vi "Rozdziel_na_Syg_typ.vi"(6 "Property Syg_typ":string[](array[string]), 8 "error in (no error)":errorcluster, 9 "data":waveform(dbl)[](array[waveform])) -> (0 "error out":errorcluster, 3 "Przebiegi":T1)   [LabVIEW 2014]
doc: "Rozdziela przebiegi wczytane z pliku TDMS\nna typy Analogowy, Cyfrowy i enkoderowy\ndla okna edycji, zgodnie z typedef Kanaly.ctl"
uses:
  Kontrolki/Przetwarzanie/Kanaly.ctl
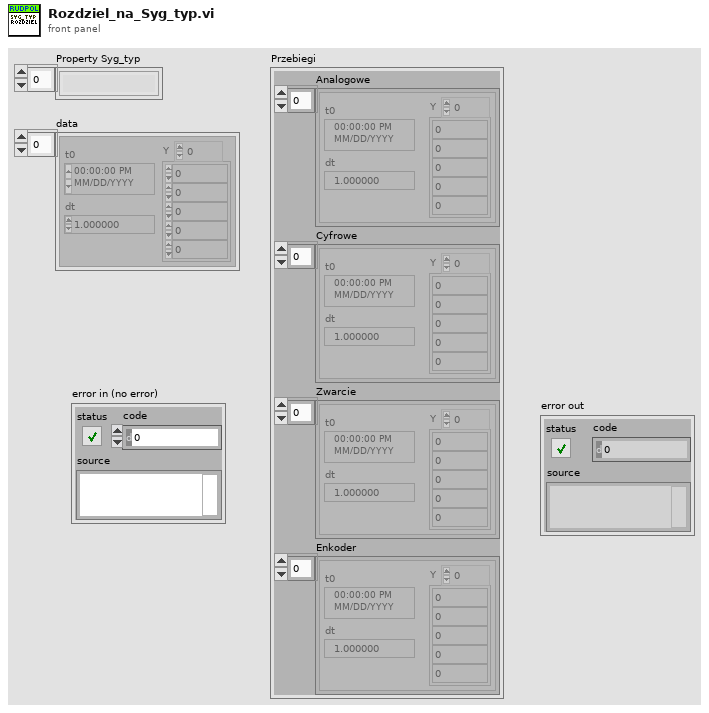
[diagram p1: front panel]
types:
  T1 = typedef "Kanaly.ctl" = cluster{"Analogowe":waveform(dbl)[], "Cyfrowe":waveform(dbl)[], "Zwarcie":waveform(dbl)[], "Enkoder":waveform(dbl)[]}
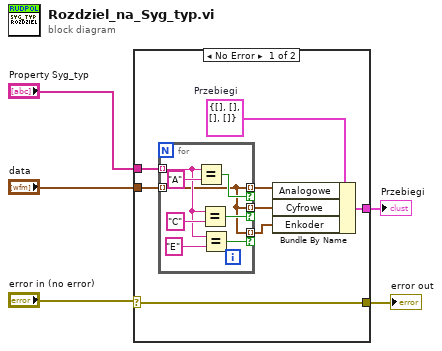
[diagram p0: block diagram]
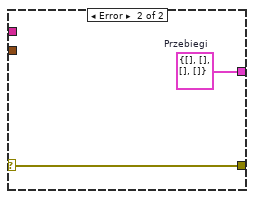
[diagram p2: hidden frame]
diagram:
  n1 = case shown="No Error" "error in (no error)" {
    selector: "error in (no error)" -> [w6 w22]
    tunnel: [w13 w23] -> w5
    tunnel: "data" -> [w8 _]
    tunnel: "Property Syg_typ" -> [w7 _]
    tunnel: [w6 w22] -> w1
    frame No Error {
      w11 = T1 {"Analogowe"=[], "Cyfrowe"=[], "Zwarcie"=[], "Enkoder"=[]}  # Przebiegi
      n2 = for {
        tunnel: w7 -> [w16] mode=indexing
        tunnel: w8 -> [w15] mode=indexing
        tunnel: [w15] -> w9 mode=indexing if=w18
        tunnel: [w15] -> w10 mode=indexing if=w17
        tunnel: [w15] -> w12 mode=indexing if=w14
        n3 = Equal?(x=w16, y="A") -> (x = y?=w18:bool)
        n4 = Equal?(x=w16, y="C") -> (x = y?=w17:bool)
        n5 = Equal?(x=w16, y="E") -> (x = y?=w14:bool)
      }
      n6 = Bundle By Name(cluster=w11, "Analogowe"=w9, "Cyfrowe"=w10, "Enkoder"=w12) -> (w13:T1)
    }
    frame Error {
      w23 = T1 {"Analogowe"=[], "Cyfrowe"=[], "Zwarcie"=[], "Enkoder"=[]}  # Przebiegi
    }
  }
  "Przebiegi" <- w5
  "error out" <- w1
